vi "Mod_OFDM_check_Status.vi"(0 "Configuration in":variant, 11 "error in":errorcluster) -> (4 "Configuration out":variant, 14 "Status":T1, 15 "error out":errorcluster)   [LabVIEW 2010]
doc: "This is a cluster of indicators to display the current configuration status. It contains following information:\n\n1. Pool Size (Data source): Displays the number of Data sources that have been configured. \n\n2. Pool Size (Modulator source): Displays the number of Modulator sources that have been configured. \n\n3. OFDM Symbol? The indicator is set to TRUE, if at lease one OFDM symbol has been configured.\n\n Sub Carrier: Displays total number of sub carriers in the current OFDM Symbol\n\n Cyclic Prefix: Displays number of sample that will be used for Cyclic Prefix\n\n4. OFDM Frame? The indicator is set to TRUE if at lease one OFDM symbol has been included in the OFDM Frame. \n\n5. Transmit Filter: This displays the filter selected in Step 5 for pulse shaping."
uses:
  Polymorphic_Sub_VI's/Mod_OFDM_Get_Data_Sources.vi
  Polymorphic_Sub_VI's/Mod_OFDM_Get_Modulator_Sources.vi
  Polymorphic_Sub_VI's/Mod_OFDM_Get_OFDM_Frame.vi
  Polymorphic_Sub_VI's/Mod_OFDM_Get_Pulse_Shaping.vi
  Polymorphic_Sub_VI's/Mod_OFDM_Get_Ofdm_Parameters.vi
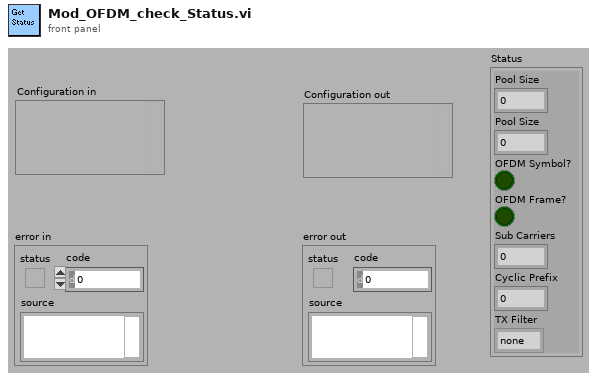
[diagram p1: front panel]
types:
  T1 = cluster{"Pool Size":i32, "Pool Size":i32, "OFDM Symbol?":bool, "OFDM Frame?":bool, "Sub Carriers":i32, "Cyclic Prefix":i32, "TX Filter":enum16{"none", "Raised Cosine", "Root Raised Cos"}}
  T2 = enum16{"none", "Raised Cosine", "Root Raised Cos"}
  T3 = cluster{"# of Sub Carrier":i32, "Length Of Cylic Prefix":i32}
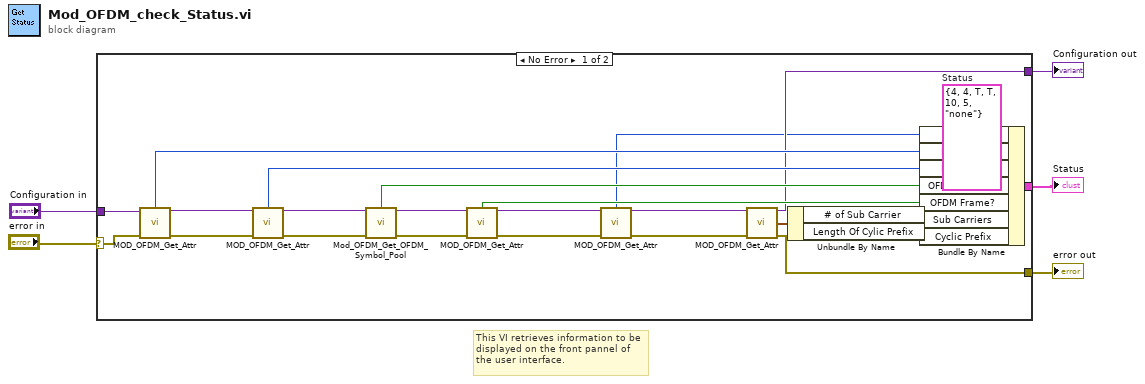
[diagram p0: block diagram]
diagram:
  # "This VI retrieves information to be displayed on the front pannel of the user interface."
  n1 = case shown="No Error" "error in" {
    selector: "error in" -> [w27 w30]
    tunnel: [w23 w30] -> w3
    tunnel: "Configuration in" -> [w28 _]
    tunnel: [w13 _] -> w2
    tunnel: [w12 _] -> w1
    frame No Error {
      w9 = T1 {"Pool Size"=4, "Pool Size"=4, "OFDM Symbol?"=TRUE, "OFDM Frame?"=TRUE, "Sub Carriers"=10, "Cyclic Prefix"=5, "TX Filter"=enum."none"}  # Status
      n2 = call-poly "MOD_OFDM_Get_Attr.vi"("Configuration in"=w28, "error in"=w27) -> ("# of Data Sources"=w19:i32, "Configuration out"=w22:variant, "error out"=w26:errorcluster)  [unwired: 7 in, 4 out]
      n3 = call-poly "MOD_OFDM_Get_Attr.vi"("Configuration in"=w22, "error in"=w26) -> ("# of Modulators"=w18:i32, "Configuration out"=w21:variant, "error out"=w25:errorcluster)  [unwired: 8 in, 3 out]
      n4 = call-poly "Mod_OFDM_Get_OFDM_Symbol_Pool.vi"("Configuration in"=w21, "error in"=w25) -> ("Symbol Status"=w17:bool, "Configuration out"=w20:variant, "error out"=w24:errorcluster)  [unwired: 8 in, 3 out]
      n5 = call-poly "MOD_OFDM_Get_Attr.vi"("Configuration in"=w20, "error in"=w24) -> ("Frame Status"=w16:bool, "Configuration out"=w10:variant, "error out"=w11:errorcluster)  [unwired: 10 in, 1 out]
      n6 = call-poly "MOD_OFDM_Get_Attr.vi"("Configuration in"=w10, "error in"=w11) -> ("TX Filter"=w6:T2, "Configuration out"=w8:variant, "error out"=w7:errorcluster)  [unwired: 10 in, 1 out]
      n7 = call-poly "MOD_OFDM_Get_Attr.vi"("Configuration in"=w8, "error in"=w7) -> ("Configuration out"=w12:variant, "OFDM Parameters"=w29:T3, "error out"=w23:errorcluster)  [unwired: 10 in, 1 out]
      n8 = Unbundle By Name(w29) -> ("# of Sub Carrier"=w15:i32, "Length Of Cylic Prefix"=w14:i32)
      n9 = Bundle By Name(cluster=w9, "TX Filter"=w6, "Pool Size"=w19, "Pool Size"=w18, "OFDM Symbol?"=w17, "OFDM Frame?"=w16, "Sub Carriers"=w15, "Cyclic Prefix"=w14) -> (w13:T1)
    }
    frame Error {
    }
  }
  "error out" <- w3
  "Configuration out" <- w1
  "Status" <- w2
